vi "Diff_Drive_System_Acquire.vi"(6 "FPGA_Time_Seconds":dbl, 11 "DiffDriveDeviceRefs":T1 {"GyroDevRef"."Sample Rate" min=0.25 max=100.0 step=0.25}) -> (2 "Right Speed":dbl, 3 "Left Speed":dbl)   [LabVIEW 2019]
uses:
  Diff_Drive_System_Device_Refs.ctl
  <vilib>/Rock Robotics/WPI/Gyro/WPI_GyroDevRef.ctl
  <vilib>/Rock Robotics/SystemInterfaces/AI/FPGA_AIChannel.ctl
  <vilib>/Rock Robotics/SystemInterfaces/spilib/spi_bus.ctl
  <vilib>/Rock Robotics/WPI/RobotDrive/WPI_RobotDriveDevRef.ctl
  <vilib>/Rock Robotics/WPI/MotorControl/WPI_MotorControlDeviceRef.ctl
  <vilib>/Rock Robotics/WPI/MotorControl/WPI_MotorControlType.ctl
  <vilib>/Rock Robotics/SystemInterfaces/DIO/FPGA_DIOPWMChannel.ctl
  <vilib>/Rock Robotics/WPI/PWM/WPI_PWMDeadband.ctl
  <vilib>/Rock Robotics/SystemInterfaces/DIO/FPGA_DIOChannel.ctl
  <vilib>/Rock Robotics/WPI/Encoder/WPI_EncoderDevRef.ctl
  <vilib>/Rock Robotics/SystemInterfaces/Encoder/FPGA_EncoderIdx.ctl
  <vilib>/Rock Robotics/SystemInterfaces/Counter/FPGA_CounterCtrSystemIndex.ctl
  <vilib>/Rock Robotics/WPI/Encoder/WPI_EncoderType.ctl
  <vilib>/Rock Robotics/SystemInterfaces/AI/FPGA_AIGyroChannel.ctl
  <vilib>/Rock Robotics/WPI/ThirdParty/JAS_Junk/TrajLib/LinearFilter_ResetToValue.vi
  <vilib>/Rock Robotics/WPI/ThirdParty/JAS_Junk/TrajLib/LinearFilter_Calculate.vi
  Diff_Drive_System_Globals.vi
  <vilib>/Rock Robotics/WPI/ThirdParty/JAS_Junk/TrajLib/LinearFilter_MovingAverage.vi
  <vilib>/Rock Robotics/WPI/ThirdParty/JAS_Junk/TrajLib/LinearFilter_LowPassBW1.vi
  <vilib>/Rock Robotics/WPI/ThirdParty/JAS_Junk/TrajLib/LinearFilter_LowPassBW2.vi
  <vilib>/Rock Robotics/WPI/ThirdParty/JAS_Junk/TrajLib/LinearFilter_HighPassBW1.vi
  <vilib>/Rock Robotics/WPI/ThirdParty/JAS_Junk/TrajLib/LinearFilter_HighPassBW2.vi
  <vilib>/Rock Robotics/WPI/ThirdParty/JAS_Junk/TrajLib/Trajectory_Library.lvlib
panel:
  # "Analog"
  # "XRS"
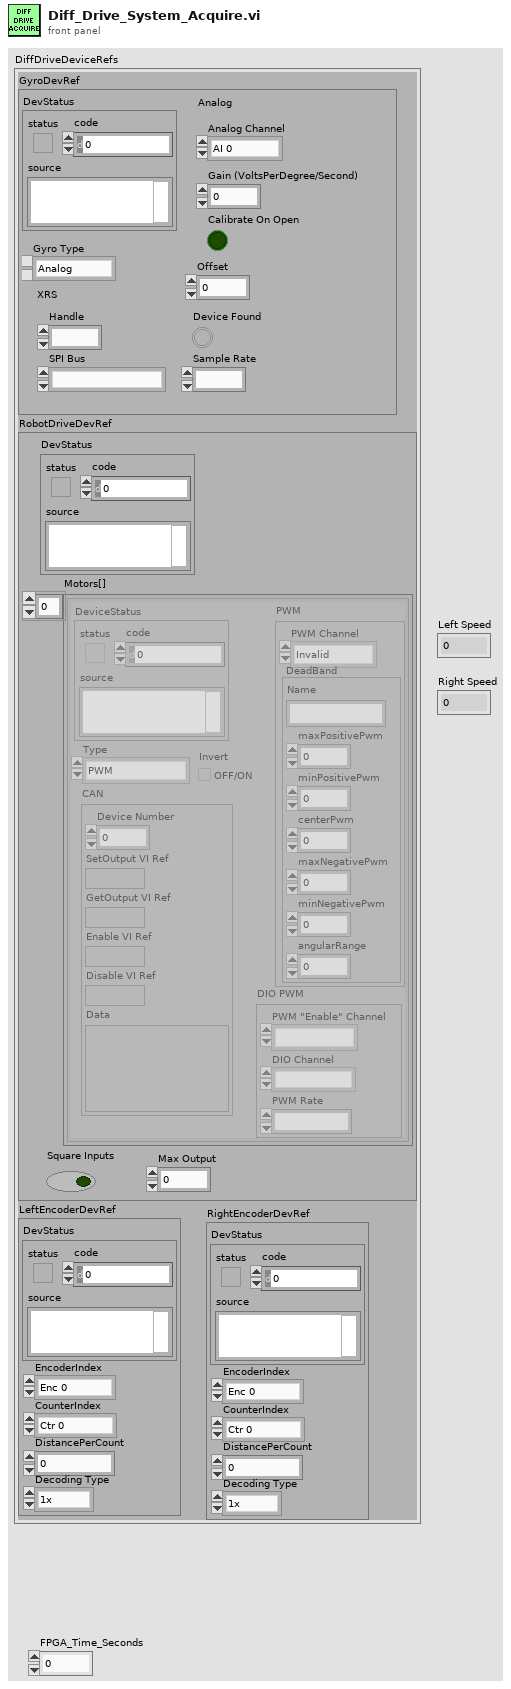
[diagram p1: front panel]
types:
  T1 = typedef "Diff_Drive_System_Device_Refs.ctl" = cluster{"GyroDevRef":T2, "RobotDriveDevRef":T5, "LeftEncoderDevRef":T11, "RightEncoderDevRef":T11}
  T2 = typedef "WPI_GyroDevRef.ctl" = cluster{"DevStatus":errorcluster, "Analog Channel":T3, "Gain (VoltsPerDegree/Second)":dbl, "Gyro Type":enum16{"Analog", "XRS450"}, "Handle":i32, "SPI Bus":T4, "Device Found":bool, "Sample Rate":dbl, "Calibrate On Open":bool, "Offset":dbl}
  T3 = typedef "FPGA_AIChannel.ctl" = enum8{"AI 0", "AI 1", "AI 2", "AI 3", "AI MXP 0", "AI MXP 1", "AI MXP 2", "AI MXP 3", "Invalid"}
  T4 = typedef "spi_bus.ctl" = enum16{"SPI On-Board, CS0", "SPI On-Board, CS1", "SPI On-Board, CS2", "SPI On-Board, CS3", "SPI MXP", "Invalid"}
  T5 = typedef "WPI_RobotDriveDevRef.ctl" = cluster{"DevStatus":errorcluster, "Motors[]":T6[], "Square Inputs":bool, "Max Output":dbl}
  T6 = typedef "WPI_MotorControlDeviceRef.ctl" = cluster{"DeviceStatus":errorcluster, "Type":T7, "PWM":cluster{"PWM Channel":T8, "DeadBand":T9}, "CAN":cluster{"Device Number":u8, "SetOutput VI Ref":variant, "GetOutput VI Ref":variant, "Enable VI Ref":variant, "Disable VI Ref":variant, "Data":variant}, "Invert":bool, "DIO PWM":cluster{"PWM \"Enable\" Channel":T8, "DIOChannel":T10, "PWM Rate":dbl}}
  T7 = typedef "WPI_MotorControlType.ctl" = enum16{"PWM", "CAN", "DIO PWM"}
  T8 = typedef "FPGA_DIOPWMChannel.ctl" = enum8{"PWM 0", "PWM 1", "PWM 2", "PWM 3", "PWM 4", "PWM 5", "PWM 6", "PWM 7", "PWM 8", "PWM 9", "PWM MXP 0", "PWM MXP 1", "PWM MXP 2", "PWM MXP 3", "PWM MXP 4", "PWM MXP 5", "PWM MXP 6", "PWM MXP 7", "PWM MXP 8", "PWM MXP 9", "Invalid"}
  T9 = typedef "WPI_PWMDeadband.ctl" = cluster{"Name":string, "maxPositivePwm":i32, "minPositivePwm":i32, "centerPwm":i32, "maxNegativePwm":i32, "minNegativePwm":i32, "angularRange":u16}
  T10 = typedef "FPGA_DIOChannel.ctl" = enum8{"DIO 0", "DIO 1", "DIO 2", "DIO 3", "DIO 4", "DIO 5", "DIO 6", "DIO 7", "DIO 8", "DIO 9", "DIO MXP 0", "DIO MXP 1", "DIO MXP 2", "DIO MXP 3", "DIO MXP 4", "DIO MXP 5", "DIO MXP 6", "DIO MXP 7", "DIO MXP 8", "DIO MXP 9", "DIO MXP 10", "DIO MXP 11", "DIO MXP 12", "DIO MXP 13", "DIO MXP 14", "DIO MXP 15", "SPI Port CS1", "SPI Port CS2", "SPI Port CS3", "SPI Port MISO", "SPI Port MOSI", "Invalid"}
  T11 = typedef "WPI_EncoderDevRef.ctl" = cluster{"DevStatus":errorcluster, "EncoderIndex":T12, "CounterIndex":T13, "DistancePerCount":dbl, "Decoding Type":T14}
  T12 = typedef "FPGA_EncoderIdx.ctl" = enum8{"Enc 0", "Enc 1", "Enc 2", "Enc 3", "Enc 4", "Enc 5", "Enc 6", "Enc 7", "Invalid"}
  T13 = typedef "FPGA_CounterCtrSystemIndex.ctl" = enum8{"Ctr 0", "Ctr 1", "Ctr 2", "Ctr 3", "Ctr 4", "Ctr 5", "Ctr 6", "Ctr 7", "Invalid"}
  T14 = typedef "WPI_EncoderType.ctl" = enum16{"1x", "2x", "4x"}
  T15 = enum16{"Moving Average", "Low Pass 1st Order Butterworth", "Low Pass 2nd Order Butterworth", "High Pass 1st Order Butterworth", "High Pass 2nd Order Butterworth"}
  T16 = typedef "FPGA_AIGyroChannel.ctl" = enum8{"AI 0", "AI 1", "Invalid"}
  T17 = cluster{">angleX":dbl, ">angleY":dbl, ">angleZ":dbl}
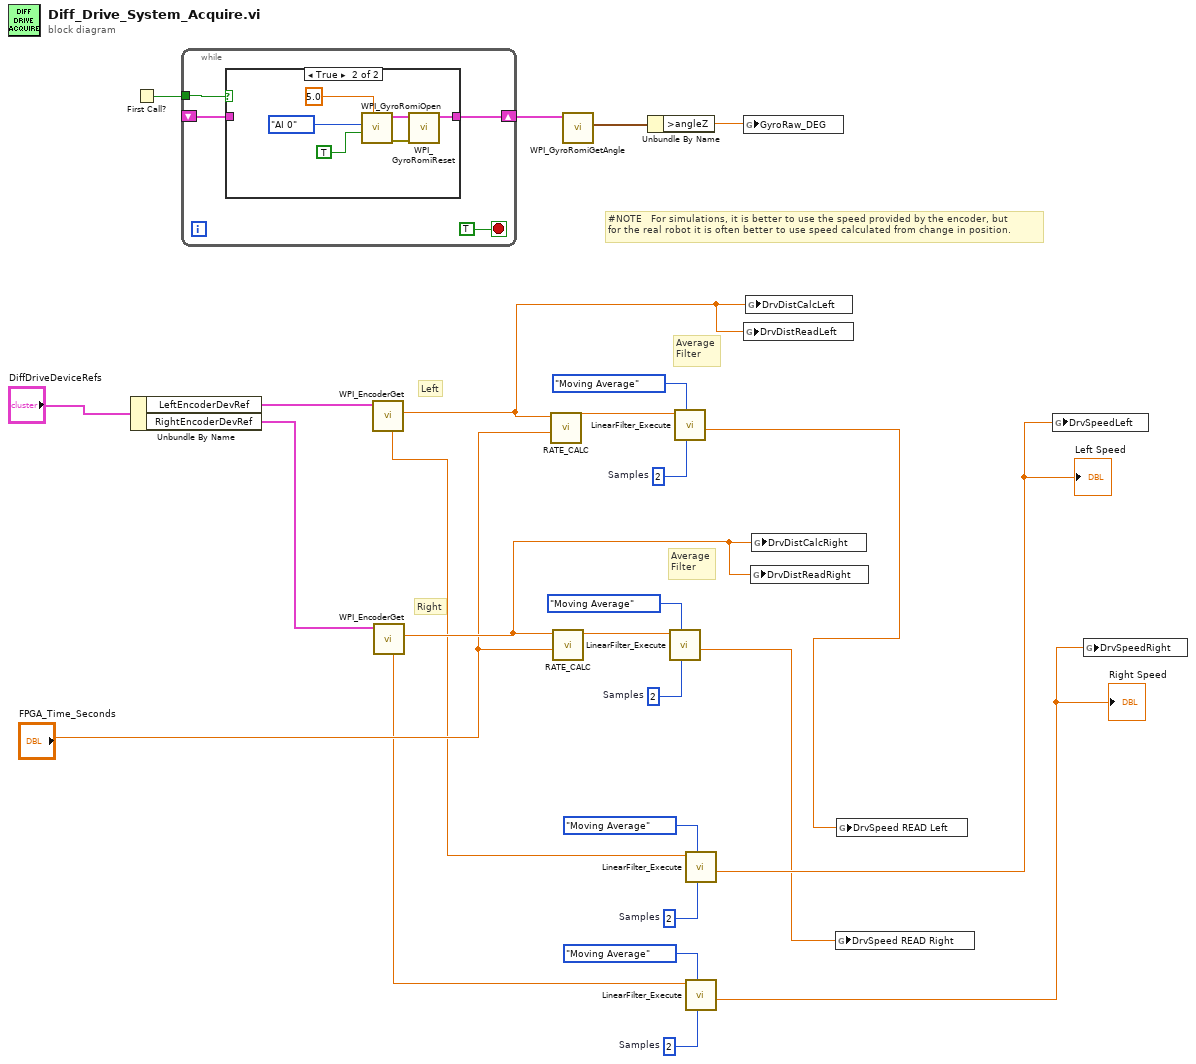
[diagram p0: block diagram]
diagram:
  w8 = 2  # Samples
  w10 = 2  # Samples
  w13 = 2  # Samples
  w16 = 2  # Samples
  # "#NOTE   For simulations, it is better to use the speed provided by the encoder, but\nfor the real robot it is often better to use speed calculated from change in position."
  # "Average\nFilter"
  # "Average\nFilter"
  # "Right"
  # "Left"
  n1 = Unbundle By Name("DiffDriveDeviceRefs") -> ("LeftEncoderDevRef"=w25:T11, "RightEncoderDevRef"=w24:T11)
  n2 = First Call?() -> (First Call?: T/F=w23:bool)
  n3 = while {
    tunnel: w23 -> [w30]
    shift-right: [w28] -> w22
    shift-left: _ -> [w27]
    stop <- TRUE stop-if-true
    n4 = case shown="True" w30 {
      tunnel: [w31 w32] -> w28
      tunnel: w27 -> [w31 _]
      frame False {
      }
      frame True {
        n5 = call <vilib>:"WPI_GyroRomiOpen.vi"("Calibration Time (s)"=5.0, "Calibrate On Open"=TRUE, "Analog Channel"=FPGA_AIGyroChannel."AI 0") -> ("error out"=w34:errorcluster, "GyroDevRef"=w33:T2)  [unwired: 7 in]
        n6 = call <vilib>:"WPI_GyroRomiReset.vi"("error in (no error)"=w34, "GyroDevRef"=w33) -> ("GyroDevRef"=w32:T2)  [unwired: 8 in, 1 out]
      }
    }
  }
  n7 = call <vilib>:"WPI_EncoderGet.vi"("EncoderDevRef"=w25) -> ("Distance"=w19:dbl, "Rate"=w6:dbl)  [unwired: 5 in, 4 out]
  n8 = call <vilib>:"WPI_EncoderGet.vi"("EncoderDevRef"=w24) -> ("Distance"=w18:dbl, "Rate"=w5:dbl)  [unwired: 5 in, 4 out]
  n9 = call "RATE_CALC.vi"("Time"="FPGA_Time_Seconds", "Input"=w19) -> ("Output"=w14:dbl)  [unwired: 9 in]
  n10 = call "RATE_CALC.vi"("Time"="FPGA_Time_Seconds", "Input"=w18) -> ("Output"=w11:dbl)  [unwired: 9 in]
  n11 = call <vilib>:"WPI_GyroRomiGetAngle.vi"("GyroDevRef"=w22) -> ("Angle"=w21:T17)  [unwired: 6 in, 4 out]
  n12 = Unbundle By Name(w21) -> (">angleZ"=w20:dbl)
  n13 = call <vilib>:"LinearFilter_Execute.vi"("Samples"=w13, "Filter Type"=T15."Moving Average", "Input"=w11) -> ("Output"=w1:dbl)  [unwired: 7 in, 1 out]
  n14 = call <vilib>:"LinearFilter_Execute.vi"("Samples"=w16, "Filter Type"=T15."Moving Average", "Input"=w14) -> ("Output"=w2:dbl)  [unwired: 7 in, 1 out]
  n15 = call <vilib>:"LinearFilter_Execute.vi"("Samples"=w10, "Filter Type"=T15."Moving Average", "Input"=w6) -> ("Output"=w4:dbl)  [unwired: 7 in, 1 out]
  "Left Speed" <- w4
  n16 = call <vilib>:"LinearFilter_Execute.vi"("Samples"=w8, "Filter Type"=T15."Moving Average", "Input"=w5) -> ("Output"=w3:dbl)  [unwired: 7 in, 1 out]
  "Right Speed" <- w3
  n17 = global write "Diff_Drive_System_Globals.vi" "GyroRaw_DEG"(w20) -> ()
  n18 = global write "Diff_Drive_System_Globals.vi" "DrvDistReadLeft"(w19) -> ()
  n19 = global write "Diff_Drive_System_Globals.vi" "DrvDistCalcLeft"(w19) -> ()
  n20 = global write "Diff_Drive_System_Globals.vi" "DrvDistReadRight"(w18) -> ()
  n21 = global write "Diff_Drive_System_Globals.vi" "DrvDistCalcRight"(w18) -> ()
  n22 = global write "Diff_Drive_System_Globals.vi" "DrvSpeed READ Right"(w1) -> ()
  n23 = global write "Diff_Drive_System_Globals.vi" "DrvSpeed READ Left"(w2) -> ()
  n24 = global write "Diff_Drive_System_Globals.vi" "DrvSpeedLeft"(w4) -> ()
  n25 = global write "Diff_Drive_System_Globals.vi" "DrvSpeedRight"(w3) -> ()
